vi "allgo 5.vi"(7 "error in":errorcluster) -> ()   [LabVIEW 2015]
uses:
  <vilib>/vision/Measure.llb/Edge Options.ctl
  <vilib>/vision/Measure.llb/Edge Polarity.ctl
  <vilib>/vision/driver/NI_Vision_Acquisition_Software.lvlib
  <vilib>/vision/NI_Vision_Development_Module.lvlib
panel:
  out "error out":errorcluster
  out "Fitted Circle":T1 {"Average SNR (dB)" format="%.2f"; "Average Strength" format="%.2f"; "Roundness (Real-World)" format="%.2f"; "Radius (Real-World)" format="%.2f"; "Center (Real-World)"."Y" format="%.2f"; "Center (Real-World)"."X" format="%.2f"; "Radius (Pixels)" format="%.2f"; "Center (Pixels)"."Y" format="%.2f"; "Center (Pixels)"."X" format="%.2f"}
  out "Circles":T2(array[cluster]) {"Position"."Y" format="%.2f"; "Position"."X" format="%.2f"}
  out "Image Out":T3(plugin-control)
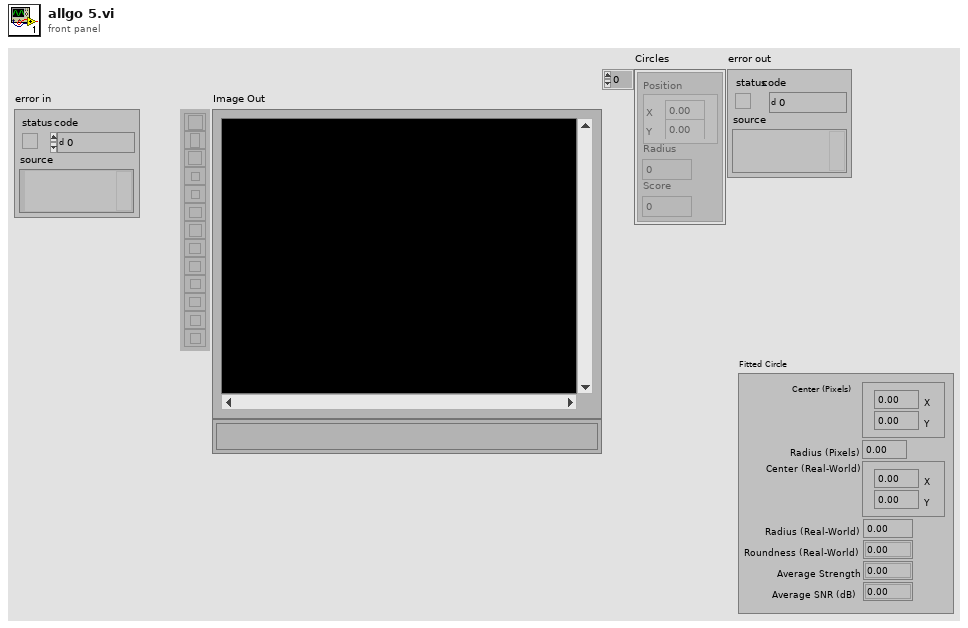
[diagram p1: front panel]
types:
  T1 = cluster{"Center (Pixels)":cluster{"X":sgl, "Y":sgl}, "Radius (Pixels)":dbl, "Center (Real-World)":cluster{"X":sgl, "Y":sgl}, "Radius (Real-World)":dbl, "Roundness (Real-World)":dbl, "Average Strength":dbl, "Average SNR (dB)":dbl}
  T2 = cluster{"Position":cluster{"X":sgl, "Y":sgl}, "Radius":dbl, "Score":dbl}[]
  T3 = typedef "IMAQ Image.ctl" = refnum<image>
  T4 = typedef "Edge Options.ctl" = cluster{"Edge Polarity":T5, "Kernel Size":u32, "Width":u32, "Minimum Edge Strength":sgl, "Interpolation Type":enum32{"Zero Order", "Bilinear", "Quadratic", "Cubic", "Bilinear Fixed"}, "Data Processing Method":enum32{"Average", "Median"}}
  T5 = typedef "Edge Polarity.ctl" = u32
  T6 = cluster{"Search  Direction":u32, "Edge Options":T4, "Show Search Area":bool, "Show Search Lines":bool, "Show Edges Found":bool, "Show Result":bool, "Search Area Color":u32, "Search Lines Color":u32, "Edge Locations Color":u32, "Result Color":u32, "Overlay Group Name":string}
  T7 = cluster{"Process":enum16{"Get First Edge", "Get First + Last Edge", "Get All Edges", "Get Best Edge"}, "Step Size":i32, "Max Pixel Radius":i32}
  T8 = cluster{"Global Rectangle":i32[], "Contours":cluster{"ID":enum32{"External", "Internal"}, "Type":u32, "Coordinates":i32[]}[]}
  T9 = cluster{"Extraction Mode":u32, "Edge Threshold":i32, "Edge Filter Size":u32, "Min Length":i32, "Row Search Step Size":i32, "Col Search Step Size":i32, "Max Endpoint Gap":i32, "Closed":bool, "Subpixel":bool}
  T10 = cluster{"Rotation":bool, "Scale":bool, "Occlusion":bool, "Range Settings":cluster{"Match Constraints":u32, "Min":dbl, "Max":dbl}[]}
  T11 = typedef "IMAQdx.ctl" = refnum<k21>
  T12 = typedef "Image Type" = u32
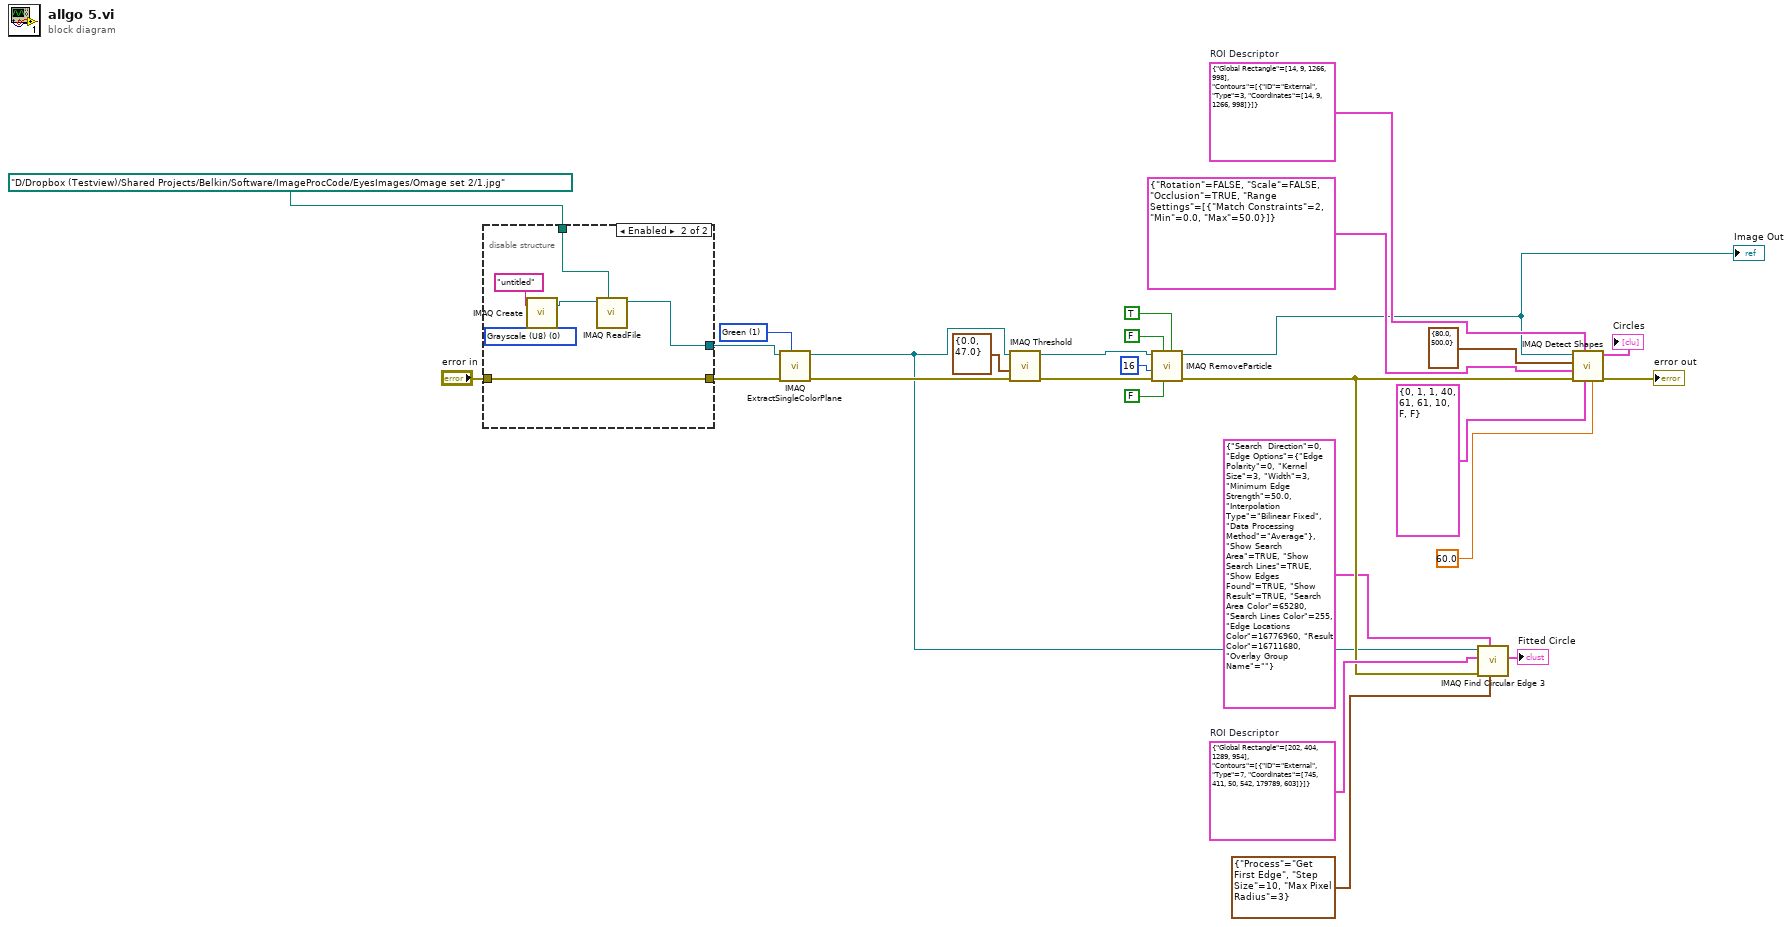
[diagram p0: block diagram]
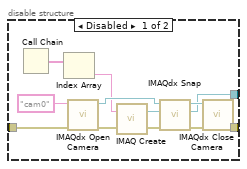
[diagram p2: hidden frame]
diagram:
  w11 = T8 {"Global Rectangle"=[202, 404, 1289, 954], "Contours"=[{"ID"=enum."External", "Type"=7, "Coordinates"=[745, 411, 50, 542, 179789, 603]}]}  # ROI Descriptor
  w12 = T8 {"Global Rectangle"=[14, 9, 1266, 998], "Contours"=[{"ID"=enum."External", "Type"=3, "Coordinates"=[14, 9, 1266, 998]}]}  # ROI Descriptor
  w26 = 1 items=["Red", "Green", "Blue", "Hue", "Saturation", "Luminance", "Value", "Intensity"] ("Color Plane")
  n1 = disable-structure shown="Enabled" {
    disable-tunnel: "error in" -> [w32 w45]
    disable-tunnel: [w29 w44] -> w2
    disable-tunnel: [w28 w45] -> w25
    disable-tunnel: path "D:/Dropbox (Testview)/Shared Projects/Belkin/Software/ImageProcCode/EyesImages/Omage set 2/1.jpg" ("File Path") -> [_ w43]
    frame Disabled {
      n2 = Call Chain() -> (call chain=w31:string[])
      n3 = Index Array(array=w31) -> (element=w30:string)  [unwired: 1 in]
      n4 = call <vilib>:"IMAQdx Open Camera.vi"("error in"=w32, "Session In"="cam0" ("Interface Name")) -> ("error out"=w38:errorcluster, "Session Out"=w33:T11)  [unwired: 1 in, 7 out]
      n5 = call "IMAQ Create"("Image Name"=w30, "error in (no error)"=w38) -> ("New Image"=w35:T3, "error out"=w34:errorcluster)  [unwired: 2 in, 1 out]
      n6 = call <vilib>:"IMAQdx Snap.vi"("error in"=w34, "Image In"=w35, "Session In"=w33) -> ("error out"=w36:errorcluster, "Image Out"=w29:T3, "Session Out"=w37:T11)  [unwired: 6 out]
      n7 = call <vilib>:"IMAQdx Close Camera.vi"("error in"=w36, "Session In"=w37) -> ("error out"=w28:errorcluster)  [unwired: 9 out]
    }
    frame Enabled {
      w40 = T12 0 items=["Grayscale (U8)", "Grayscale (I16)", "Grayscale (SGL)", "Complex (CSG)", "RGB (U32)", "HSL (U32)", "RGB (U64)", "Grayscale (U16)"] ("Image Type")
      n8 = call "IMAQ Create"("Image Name"="untitled", "Image Type"=w40) -> ("New Image"=w42:T3)  [unwired: 3 in, 1 out]
      n9 = call "IMAQ ReadFile"("File Path"=w43, "Image"=w42) -> ("Image Out"=w44:T3)  [unwired: 5 in, 4 out]
    }
  }
  n10 = call "IMAQ ExtractSingleColorPlane"("Color Plane"=w26, "error in (no error)"=w25, "Image Src"=w2) -> ("error out"=w23:errorcluster, "Image Dst Out"=w7:T3)  [unwired: 1 in, 6 out]
  n11 = call "IMAQ Threshold"("error in (no error)"=w23, "Range"=cluster{"Lower value":sgl, "Upper value":sgl} {"Lower value"=0.0, "Upper value"=47.0}, "Image Src"=w7) -> ("error out"=w17:errorcluster, "Image Dst Out"=w18:T3)  [unwired: 3 in, 4 out]
  n12 = call "IMAQ RemoveParticle"("Connectivity 4/8 (8)"=TRUE, "Low Pass/High Pass (Low)"=FALSE, "Square/Hexa (Square)"=FALSE, "error in (no error)"=w17, "Number of Erosion"=16, "Image Src"=w18) -> ("error out"=w10:errorcluster, "Image Dst Out"=w1:T3)  [unwired: 1 in, 3 out]
  "Image Out" <- w1
  n13 = call "IMAQ Find Circular Edge 3"("Circle Fit Options"=T7 {"Process"=enum."Get First Edge", "Step Size"=10, "Max Pixel Radius"=3}, "Options"=T6 {"Search  Direction"=0, "Edge Options"={"Edge Polarity"=0, "Kernel Size"=3, "Width"=3, "Minimum Edge Strength"=50.0, "Interpolation Type"=enum."Bilinear Fixed", "Data Processing Method"=enum."Average"}, "Show Search Area"=TRUE, "Show Search Lines"=TRUE, "Show Edges Found"=TRUE, "Show Result"=TRUE, "Search Area Color"=65280, "Search Lines Color"=255, "Edge Locations Color"=16776960, "Result Color"=16711680, "Overlay Group Name"=""}, "error in (no error)"=w10, "ROI Descriptor"=w11, "Image"=w7) -> ("Fitted Circle"=→"Fitted Circle":T1)  [unwired: 2 in, 4 out]
  n14 = call-poly "IMAQ Detect Shapes"("Minimum match score"=60.0, "Curve Parameters"=T9 {"Extraction Mode"=0, "Edge Threshold"=1, "Edge Filter Size"=1, "Min Length"=40, "Row Search Step Size"=61, "Col Search Step Size"=61, "Max Endpoint Gap"=10, "Closed"=FALSE, "Subpixel"=FALSE}, "ROI Descriptor"=w12, "error in (no error)"=w10, "Match Options"=T10 {"Rotation"=FALSE, "Scale"=FALSE, "Occlusion"=TRUE, "Range Settings"=[{"Match Constraints"=2, "Min"=0.0, "Max"=50.0}]}, "Circle Descriptor"=cluster{"Min Radius":dbl, "Max Radius":dbl} {"Min Radius"=80.0, "Max Radius"=500.0}, "Image"=w1) -> ("error out"=→"error out":errorcluster, "Circles"=→"Circles":T2)  [unwired: 3 out]
